vi "Start Cooker.vi"(8 "error in (no error)":errorcluster, 9 "Duration (s)":dbl, 10 "Set Fire (%)":dbl min=0.0 max=100.0 format="%.2f %", 11 "Ramp Cooker in":refnum<class "Ramp Cooker.lvclass">) -> (0 "error out":errorcluster, 3 "Ramp Cooker out":refnum<class "Ramp Cooker.lvclass">)   [LabVIEW 2024, in "Cooker Actor.lvlib" / "Ramp Cooker.lvclass"]
uses:
  Ramp Cooker.lvclass
  Cooker Actor/Cooker Actor.lvclass
  Ramp Cooker.lvclass/Ramp Cooker.ctl
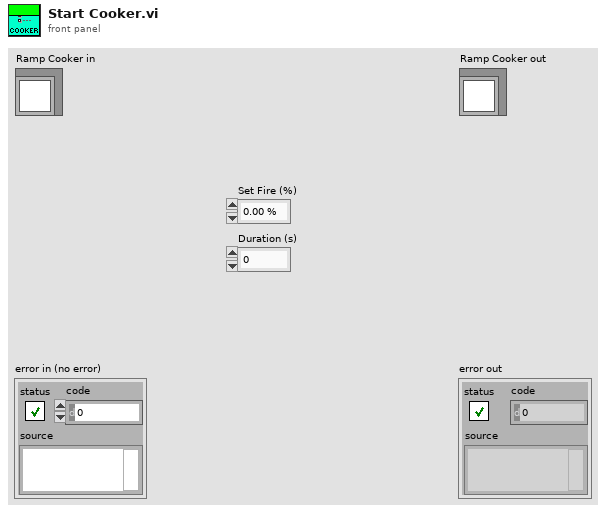
[diagram p1: front panel]
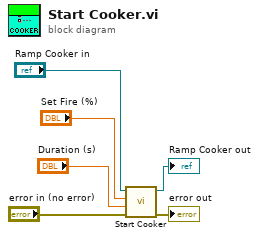
[diagram p0: block diagram]
diagram:
  n1 = call-parent "Start Cooker.vi"("error in (no error)"="error in (no error)", "Duration (s)"="Duration (s)", "Set Fire (%)"="Set Fire (%)", "Cooker Actor in"="Ramp Cooker in") -> ("error out"=→"error out":errorcluster, "Cooker Actor out"=→"Ramp Cooker out":refnum<class "Ramp Cooker.lvclass">)  [unwired: 6 in]
